vi "Version to String.vi"(11 "Version":T1) -> (3 "String":string)   [LabVIEW 2019, in "Builder.lvclass"]
uses:
  Builder.lvclass
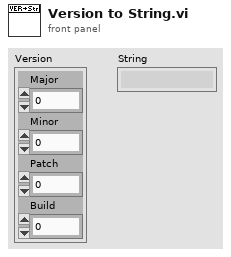
[diagram p1: front panel]
types:
  T1 = cluster{"Major":i32, "Minor":i32, "Patch":i32, "Build":i32}
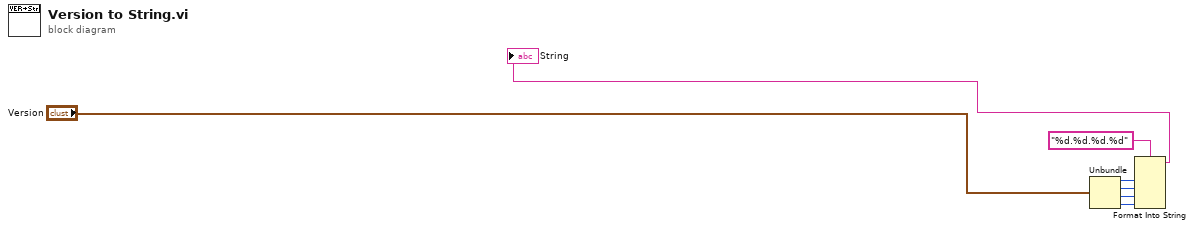
[diagram p0: block diagram]
diagram:
  n1 = Unbundle("Version") -> ("Major"=w1:i32, "Minor"=w2:i32, "Patch"=w3:i32, "Build"=w4:i32)
  n2 = Format Into String(format string="%d.%d.%d.%d", w1, w2, w3, w4) -> (resulting string=→"String":string)  [unwired: 2 in, 1 out]
